vi "random-bpm-selector.vi"(6 "Låst BPM in":i32, 9 "Lås BPM":bool, 10 "Lower BPM":i32, 11 "Upper BPM":i32) -> (3 "BPM out":i32)   [LabVIEW 2019]
uses:
  <vilib>/numeric/Random Number (Range) I64.vi
  <vilib>/numeric/sub_Random U32.vi
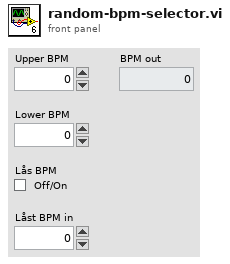
[diagram p1: front panel]
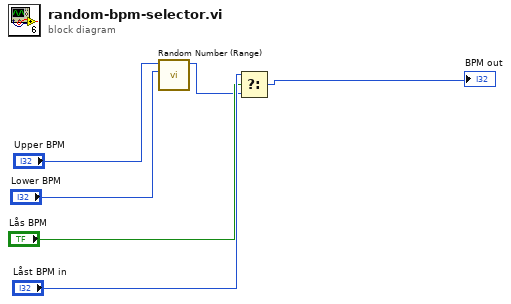
[diagram p0: block diagram]
diagram:
  n1 = call-poly <vilib>:"Random Number (Range).vi"("lower bound (-100)"="Lower BPM", "upper bound (100)"="Upper BPM") -> ("number"=w1:i64)  [unwired: 9 in]
  n2 = Select(t="Låst BPM in", s="Lås BPM", f=w1) -> (s? t:f=→"BPM out":i64)
